vi "Run Protocol.vi"(8 "error in (no error)":errorcluster, 11 "Python Protocol in":refnum<class "Python Protocol.lvclass">) -> (0 "error out":errorcluster, 3 "Python Protocol out":refnum<class "Python Protocol.lvclass">)   [LabVIEW 2012, in "Python Protocol Actor.lvlib" / "Python Protocol.lvclass"]
uses:
  Python Protocol.lvclass
  Python Protocol.lvclass/Python Protocol.ctl
  Read Code.vi
  Read Start Time.vi
  Read DVR.vi
  Read New.vi
  Read Open.vi
  Read Save.vi
  Read Refresh.vi
  Read Compiler.vi
  Read State.vi
  <userlib>/_OpenG.lib/labpython/labpython.llb/PYTHON Set Float Data__ogtk.vi
  <userlib>/_OpenG.lib/labpython/labpython.llb/PYTHON Get Float Data__ogtk.vi
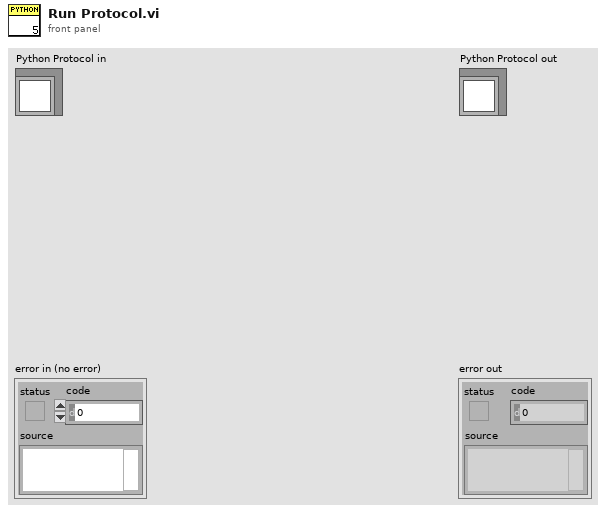
[diagram p1: front panel]
types:
  T1 = enum8{"Enabled", "Disabled", "Disabled and Grayed Out"}
  T2 = enum32{"Pause Button", "Play Button", "Media Stop Button"}
  T3 = cluster{"Name":string, "Value":dbl, "Setpoint":dbl, "Output":dbl}[]
  T4 = typedef "PYTHON Session Refnum__ogtk.ctl" = refnum<k1>
  T5 = cluster{"Name":string, "Value":dbl, "Setpoint":dbl, "Output":dbl}
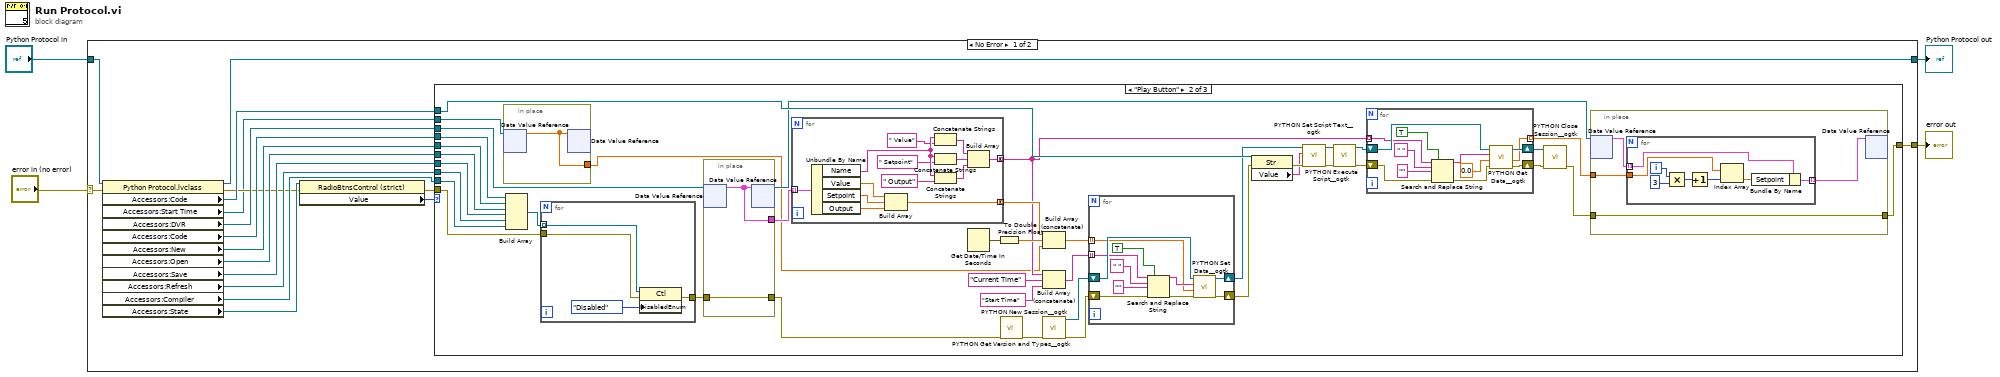
[diagram p0: block diagram]
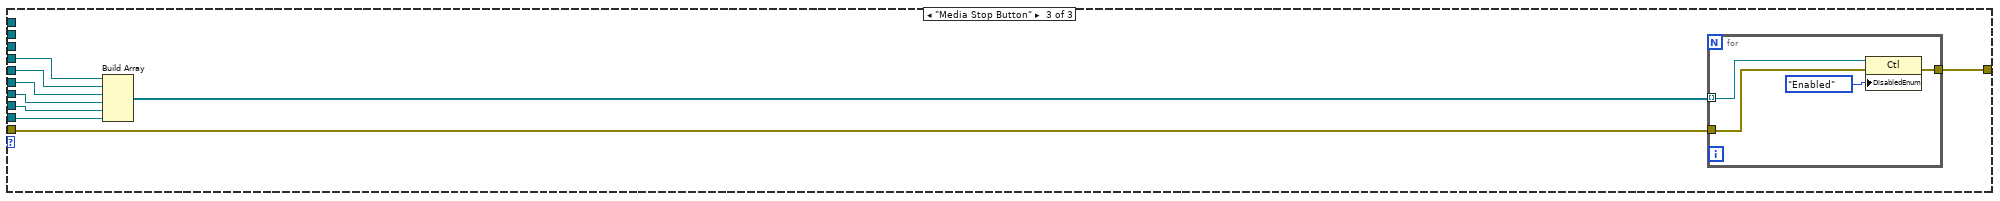
[diagram p3: hidden frame]
diagram:
  n1 = case shown="No Error" "error in (no error)" {
    selector: "error in (no error)" -> [w7 w132]
    tunnel: [w8 w132] -> w3
    tunnel: [w18 w131] -> w1
    tunnel: "Python Protocol in" -> [w19 w131]
    frame No Error {
      n2 = property class="Python Protocol.lvclass"(reference=w19, error in=w7) -> (reference out=w18:refnum<class "Python Protocol.lvclass">, error out=w6:errorcluster, "Accessors:Code"=w17:refnum<vi>, "Accessors:Start Time"=w5:refnum<data-value>, "Accessors:DVR"=w16:refnum<data-value>, "Accessors:Code"=w15:refnum<vi>, "Accessors:New"=w14:refnum<vi>, "Accessors:Open"=w13:refnum<vi>, "Accessors:Save"=w12:refnum<vi>, "Accessors:Refresh"=w11:refnum<vi>, "Accessors:Compiler"=w10:refnum<vi>, "Accessors:State"=w9:refnum<vi>)
      n3 = property class="RadioBtnsControl (strict)"(reference=w9, error in=w6) -> (error out=w21:errorcluster, "Value"=w20:T2)  [unwired: 1 out]
      n4 = case shown="\"Play Button\"" w20 {
        tunnel: w16 -> [_ w34 _]
        tunnel: [w22 w45 w118] -> w8
        tunnel: w21 -> [w22 w59 w119]
        tunnel: w10 -> [_ w54 w120]
        tunnel: w14 -> [_ w58 w124]
        tunnel: w13 -> [_ w57 w123]
        tunnel: w12 -> [_ w56 w122]
        tunnel: w11 -> [_ w55 w121]
        tunnel: w17 -> [_ w51 _]
        tunnel: w15 -> [_ w50 w125]
        tunnel: w5 -> [_ w24 _]
        frame "Pause Button", Default {
        }
        frame "Play Button" {
          n5 = in-place {
            in-place-border: [w63] -> w23
            n6 = in-place-dvr #1(w24) -> (w63:dbl)  [unwired: 1 out]
            n7 = in-place-dvr #1(w63) -> ()  [unwired: 2 out]
          }
          n8 = Build Array(w50, w58, w57, w56, w55, w54) -> (w53:refnum<vi>[])
          n9 = for {
            tunnel: w59 -> [w105]
            tunnel: [w104] -> w35
            tunnel: w53 -> [w103] mode=indexing
            n10 = property class="Ctl"(reference=w103, error in=w105, "DisabledEnum"=T1."Disabled" ("Disabled")) -> (error out=w104:errorcluster)  [unwired: 1 out]
          }
          n11 = in-place {
            in-place-border: [w78] -> w32
            in-place-border: w35 -> [w78]
            in-place-border: [w77] -> w39
            n12 = in-place-dvr #2(w34) -> (w77:T3)  [unwired: 1 out]
            n13 = in-place-dvr #2(w77) -> (w33:refnum<data-value>)  [unwired: 1 out]
          }
          n14 = for {
            tunnel: w39 -> [w76] mode=indexing
            tunnel: [w65] -> w30 mode=concatenating
            tunnel: [w64] -> w38 mode=concatenating
            n15 = Unbundle By Name(w76) -> ("Name"=w72:string, "Value"=w73:dbl, "Setpoint"=w74:dbl, "Output"=w75:dbl)
            n16 = Build Array(w73, w74, w75) -> (w64:dbl[])
            n17 = Concatenate Strings(w72, " Value" ("string")) -> (w68:string)
            n18 = Concatenate Strings(w72, " Setpoint" ("string")) -> (w67:string)
            n19 = Concatenate Strings(w72, " Output" ("string")) -> (w66:string)
            n20 = Build Array(w68, w67, w66) -> (w65:string[])
          }
          n21 = Get Date/Time In Seconds() -> (seconds since 1Jan1904=w40:timestamp)
          n22 = To Double Precision Float(number=w40) -> (double precision float=w36:dbl)
          n23 = call <userlib>:"PYTHON Get Version and Types__ogtk.vi"("error in (no error)"=w32) -> ("error out"=w62:errorcluster)  [unwired: 4 in, 2 out]
          n24 = Build Array (concatenate)(w38, w36, w23) -> (w31:dbl[])
          n25 = Build Array (concatenate)(w30, "Current Time", "Start Time" ("element")) -> (w29:string[])
          n26 = call <userlib>:"PYTHON New Session__ogtk.vi"("error in (no error)"=w62) -> ("error out"=w61:errorcluster, "Python Session"=w60:T4)  [unwired: 5 in]
          n27 = for {
            tunnel: w29 -> [w112] mode=indexing
            shift-right: [w116] -> w28
            shift-left: w60 -> [w115]
            shift-right: [w117] -> w52
            shift-left: w61 -> [w114]
            tunnel: w31 -> [w107] mode=indexing
            n28 = Search and Replace String(replace all?=TRUE ("replace all? (F)"), input string=w112, search string=" ", replace string="" ("replace string (\"\")"), error in=w114) -> (result string=w108:string, error out=w113:errorcluster)  [unwired: 3 in, 2 out]
            n29 = call-poly <userlib>:"PYTHON Set Data__ogtk.vi"("error in (no error)"=w113, "value"=w107, "variable name"=w108, "Python Session in"=w115) -> ("error out"=w117:errorcluster, "Python Session out"=w116:T4)  [unwired: 2 in]
          }
          n30 = property class="Str"(reference=w51, error in=w52) -> (error out=w27:errorcluster, "Value"=w26:string)  [unwired: 1 out]
          n31 = call <userlib>:"PYTHON Set Script Text__ogtk.vi"("error in (no error)"=w27, "script text"=w26, "Python Session in"=w28) -> ("error out"=w44:errorcluster, "Python Session out"=w43:T4)  [unwired: 3 in]
          n32 = call <userlib>:"PYTHON Execute Script__ogtk.vi"("error in (no error)"=w44, "Python Session in"=w43) -> ("error out"=w42:errorcluster, "Python Session out"=w41:T4)  [unwired: 4 in]
          n33 = for {
            tunnel: w30 -> [w97] mode=indexing
            shift-right: [w101] -> w48
            shift-left: w41 -> [w100]
            shift-right: [w102] -> w49
            shift-left: w42 -> [w99]
            tunnel: [w91] -> w46 mode=indexing
            n34 = Search and Replace String(replace all?=TRUE ("replace all? (F)"), input string=w97, search string=" ", replace string="" ("replace string (\"\")"), error in=w99) -> (result string=w93:string, error out=w98:errorcluster)  [unwired: 3 in, 2 out]
            n35 = call-poly <userlib>:"PYTHON Get Data__ogtk.vi"("error in (no error)"=w98, "data type"=0.0, "variable name"=w93, "Python Session in"=w100) -> ("error out"=w102:errorcluster, "value"=w91:dbl, "Python Session out"=w101:T4)  [unwired: 1 in]
          }
          n36 = call <userlib>:"PYTHON Close Session__ogtk.vi"("error in (no error)"=w49, "Python Session in"=w48) -> ("error out"=w47:errorcluster)  [unwired: 5 in]
          n37 = in-place {
            in-place-border: [w82] -> w45
            in-place-border: w47 -> [w82]
            in-place-border: w46 -> [w80]
            n38 = in-place-dvr #3(w33) -> (w81:T3)  [unwired: 1 out]
            n39 = for {
              tunnel: w81 -> [w90] mode=indexing
              tunnel: w80 -> [w89]
              tunnel: [w84] -> w79 mode=indexing
              i -> [w87]
              n40 = Multiply(x=w87, y=3) -> (x*y=w85:i32)
              n41 = Increment(x=w85) -> (x+1=w83:i32)
              n42 = Index Array(array=w89, index=w83) -> (element=w88:dbl)
              n43 = Bundle By Name(cluster=w90, "Setpoint"=w88) -> (w84:T5)
            }
            n44 = in-place-dvr #3(w79) -> ()  [unwired: 2 out]
          }
        }
        frame "Media Stop Button" {
          n45 = Build Array(w125, w124, w123, w122, w121, w120) -> (w126:refnum<vi>[])
          n46 = for {
            tunnel: w119 -> [w129]
            tunnel: [w128] -> w118
            tunnel: w126 -> [w127] mode=indexing
            n47 = property class="Ctl"(reference=w127, error in=w129, "DisabledEnum"=T1."Enabled" ("Disabled")) -> (error out=w128:errorcluster)  [unwired: 1 out]
          }
        }
      }
    }
    frame Error {
    }
  }
  "error out" <- w3
  "Python Protocol out" <- w1
